vi "Pump_Conditions_Check.vi"() -> (0 "OK":bool, 1 "K_Empty Out":bool, 2 "K_Closed Out":bool, 3 "P_Empty Out":bool)   [LabVIEW 2024]
panel:
  in  "Pump":bool
  in  "Ethanol":bool
  in  "Cancel Button":bool
  in  "OK Button":bool
  in  "Valve":bool
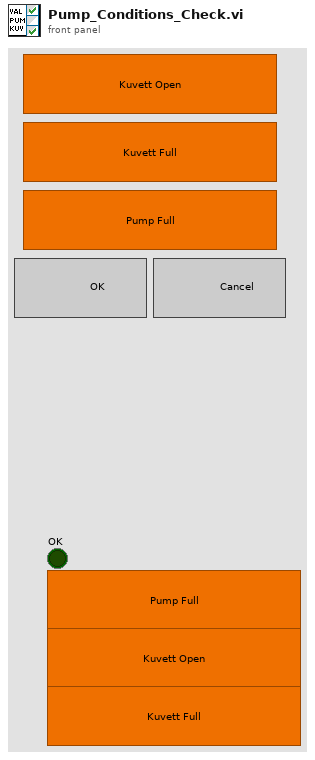
[diagram p1: front panel]
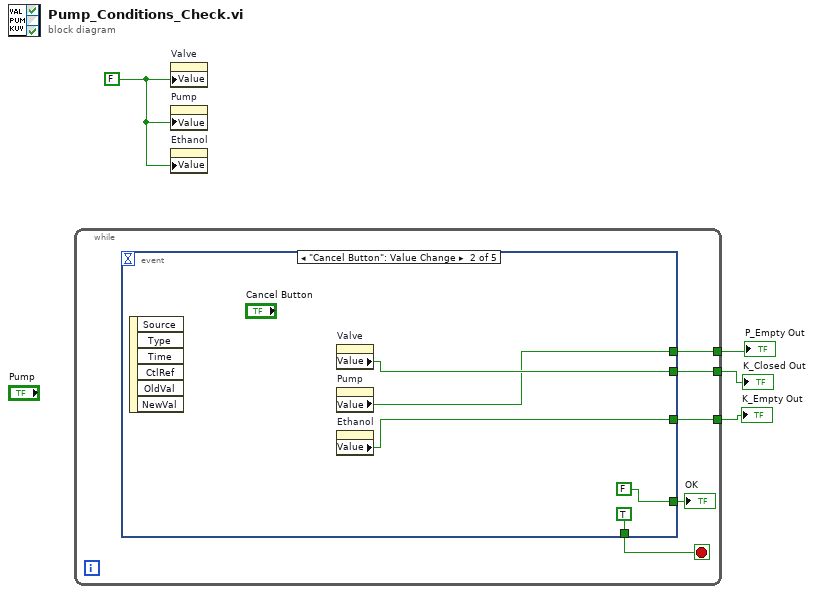
[diagram p0: block diagram]
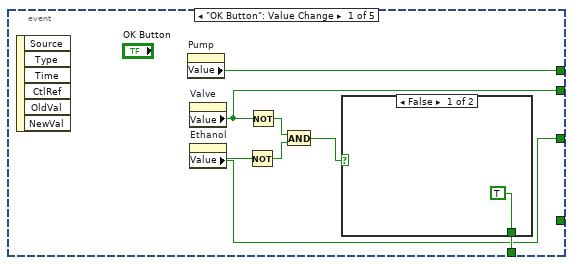
[diagram p2: hidden frame]
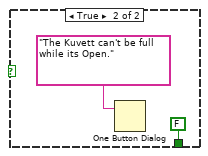
[diagram p3: hidden frame]
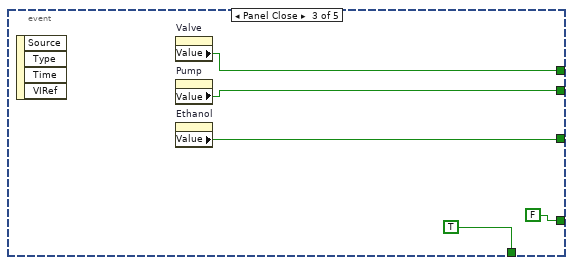
[diagram p4: hidden frame]
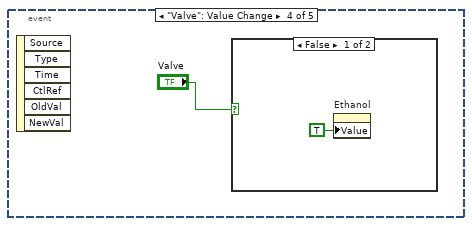
[diagram p5: hidden frame]
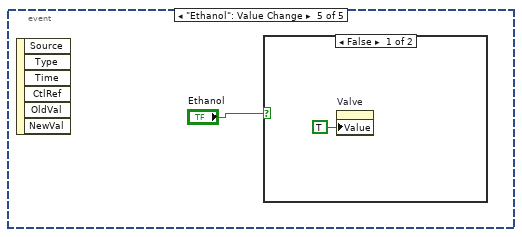
[diagram p7: hidden frame]
diagram:
  w4 = FALSE ("Valve")
  n1 = while {
    tunnel: [w8] -> w3
    tunnel: [w7] -> w2
    tunnel: [w6] -> w1
    stop <- w9 stop-if-true
    n2 = event shown="[1] \"Cancel Button\": Value Change" {
      selector: _ -> [_ _ _ _ _]
      dyn-events: _ -> [_ _ _ _ _]
      timeout: _ -> [_ _ _ _ _]
      tunnel: [w16 TRUE TRUE _ _] -> w9
      tunnel: [w12 w23 w29 _ _] -> w8
      tunnel: [w11 w24 w28 _ _] -> w7
      tunnel: [w10 w22 w27 _ _] -> w6
      tunnel: [_ FALSE ("OK") FALSE ("OK") _ _] -> w5
      event "OK Button": Value Change {
        n3 = event-data() -> ()  [unwired: 1 in, 6 out]
        n4 = property on="Pump" class="Bool (strict)"() -> ("Value"=w12:bool)  [unwired: 2 in, 2 out]
        n5 = property on="Valve" class="Bool (strict)"() -> ("Value"=w11:bool)  [unwired: 2 in, 2 out]
        n6 = property on="Ethanol" class="Bool (strict)"() -> ("Value"=w10:bool)  [unwired: 2 in, 2 out]
        n7 = Not(x=w10) -> (.not. x?=w14:bool)
        n8 = Not(x=w11) -> (.not. x?=w15:bool)
        n9 = And(x=w15, y=w14) -> (x .and. y?=w13:bool)
        n10 = case shown="False" w13 {
          tunnel: [TRUE FALSE] -> w16
          frame False {
          }
          frame True {
            n11 = One Button Dialog(message="The Kuvett can't be full while its Open.") -> ()  [unwired: 1 in, 1 out]
          }
        }
      }
      event "Cancel Button": Value Change {
        n12 = event-data() -> ()  [unwired: 1 in, 6 out]
        n13 = property on="Valve" class="Bool (strict)"() -> ("Value"=w24:bool)  [unwired: 2 in, 2 out]
        n14 = property on="Pump" class="Bool (strict)"() -> ("Value"=w23:bool)  [unwired: 2 in, 2 out]
        n15 = property on="Ethanol" class="Bool (strict)"() -> ("Value"=w22:bool)  [unwired: 2 in, 2 out]
      }
      event Panel Close {
        n16 = event-data() -> ()  [unwired: 1 in, 4 out]
        n17 = property on="Valve" class="Bool (strict)"() -> ("Value"=w29:bool)  [unwired: 2 in, 2 out]
        n18 = property on="Pump" class="Bool (strict)"() -> ("Value"=w28:bool)  [unwired: 2 in, 2 out]
        n19 = property on="Ethanol" class="Bool (strict)"() -> ("Value"=w27:bool)  [unwired: 2 in, 2 out]
      }
      event "Valve": Value Change {
        n20 = event-data() -> ()  [unwired: 1 in, 6 out]
        n21 = case shown="False" "Valve" {
          frame False {
            n22 = property on="Ethanol" class="Bool (strict)"("Value"=TRUE ("Ethanol")) -> ()  [unwired: 2 in, 2 out]
          }
          frame True {
          }
        }
      }
      event "Ethanol": Value Change {
        n23 = event-data() -> ()  [unwired: 1 in, 6 out]
        n24 = case shown="False" "Ethanol" {
          frame False {
            n25 = property on="Valve" class="Bool (strict)"("Value"=TRUE ("Valve")) -> ()  [unwired: 2 in, 2 out]
          }
          frame True {
          }
        }
      }
    }
    "OK" <- w5
  }
  "P_Empty Out" <- w3
  "K_Closed Out" <- w2
  "K_Empty Out" <- w1
  n26 = property on="Valve" class="Bool (strict)"("Value"=w4) -> ()  [unwired: 2 in, 2 out]
  n27 = property on="Pump" class="Bool (strict)"("Value"=w4) -> ()  [unwired: 2 in, 2 out]
  n28 = property on="Ethanol" class="Bool (strict)"("Value"=w4) -> ()  [unwired: 2 in, 2 out]
